vi "textParseController.vi"(8 "error in (no error)":errorcluster, 10 "file name":string, 11 "base path":path=path "C:/specsheetsController/Sheets/Controller") -> (0 "error out":errorcluster, 2 "all rows":string[][](array[string]), 3 "appended path":path)   [LabVIEW 2018]
uses:
  <vilib>/Utility/file.llb/Read Delimited Spreadsheet (string).vi
  Global textParse.vi
panel:
  out "protocolGrade":string
  out "protocolDistance":string
  out "protocolSpeed":string
  out "LED Frequency Max":string
  out "LED Frequency Min":string
  out "LED Frequency (Charge)":string
  out "LED Frequency (Limit)":string
  out "LED Frequency (Foldback)":string
  out "HV Bus Voltage(@10% PWM)":string
  out "HV Bus Tol. Min":string
  out "HV Bus Tol. Max":string
  out "Speed Pot Voltage Low(@85% PWM)":string
  out "Speed Pot Voltage Mid(@85% PWM)":string
  out "Speed Pot Voltage High(@85% PWM)":string
  out "Speed Pot Voltage Tol. Min":string
  out "Speed Pot Voltage Tol. Max":string
  out "Ircomp(@70% PWM)":string
  out "Current Running Tol. Min":string
  out "Current Running Tol. Max":string
  out "Current Limit(@45% PWM)":string
  out "Sense Voltage Tol. Max":string
  out "Sense Voltage Tol. Min":string
  out "Sense Voltage":string
  out "Allowable Power Interuption":string
  out "Voltage FET Driver Tol. Max":string
  out "Voltage FET Driver Tol. Min":string
  out "Voltage FET Driver":string
  out "Voltage Micro Tol. Max":string
  out "Voltage Micro Tol. Min":string
  out "Voltage Micro":string
  out "Rated Output Current Tol. Max":string
  out "Rated Output Current Tol. Min":string
  out "Rated Output Current":string
  out "Ripple/Noise Tol. Max":string
  out "Ripple/Noise Tol. Min":string
  out "Ripple/Noise":string
  out "Voltage Output Tol. Max":string
  out "Voltage  Output Tol. Min":string
  out "Voltage Output":string
  out "Max Input Current":string
  out "Input Current":string
  out "Input Voltage Tol. Max":string
  out "Input Voltage Tol. Min":string
  out "Input Voltage":string
  out "Firmware":string
  out "Part Number":string
  out "Part Name":string
  # "Global variables"
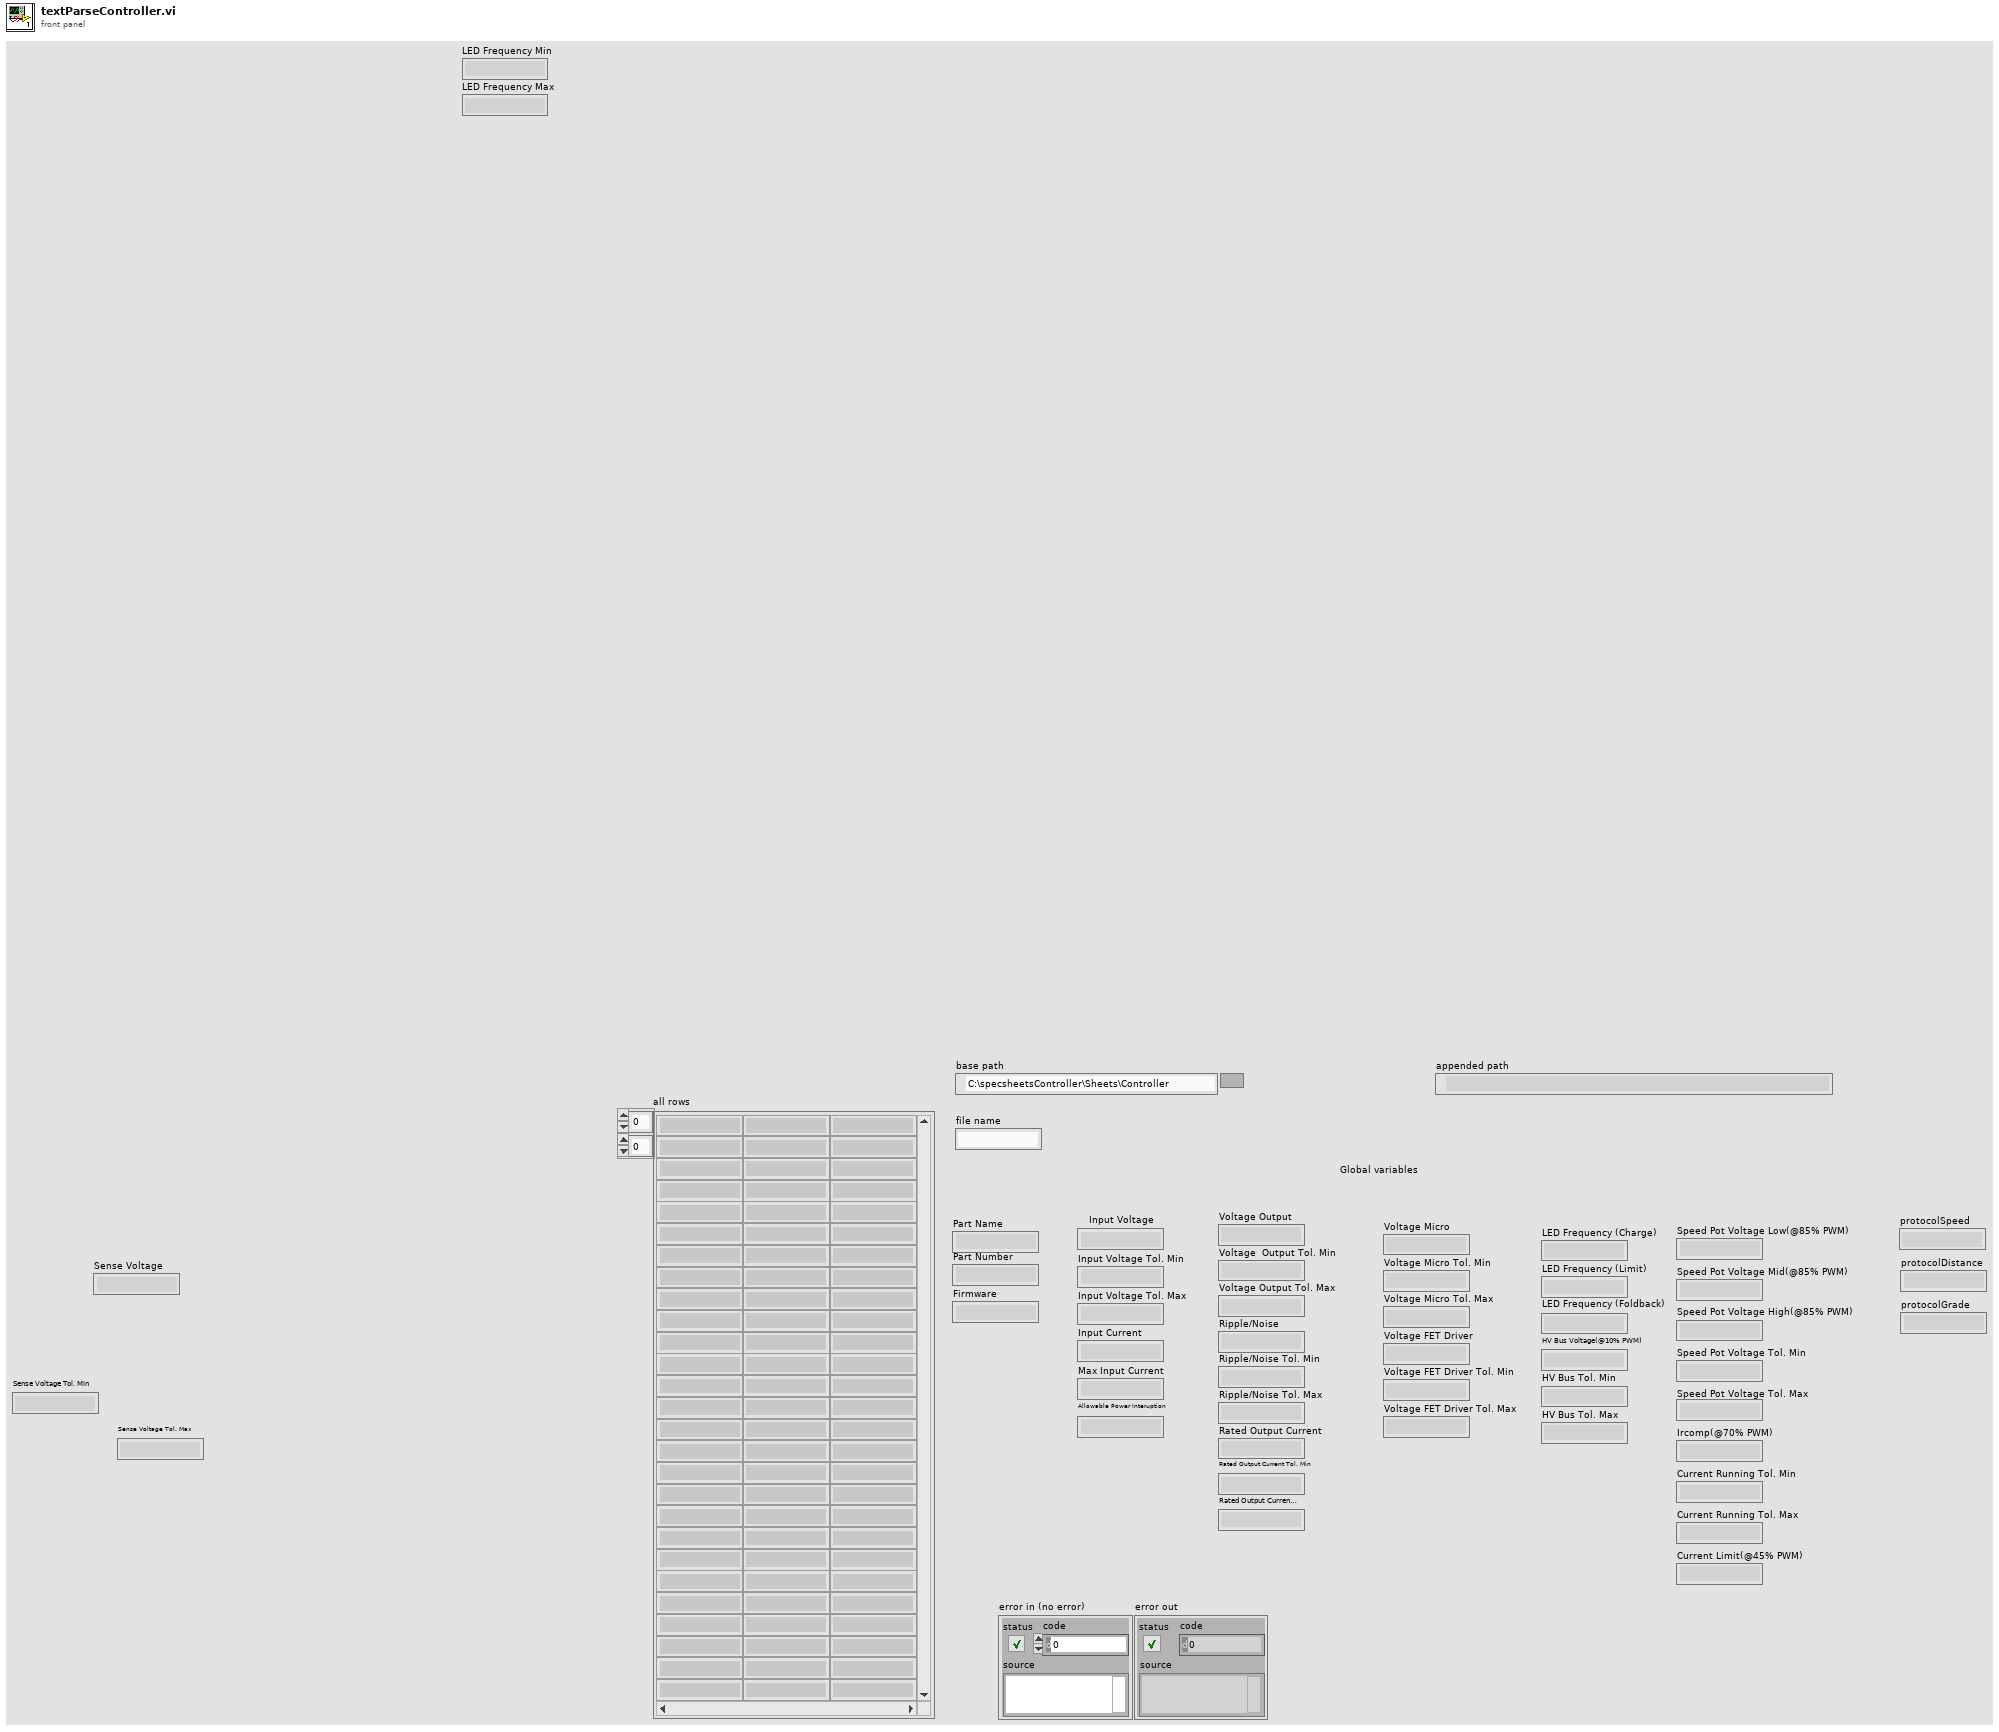
[diagram p1: front panel]
types:
  T1 = enum16{"Main", "In Primary", "Secondary", "Out Primary", "Motor Drive", "Protocol"}
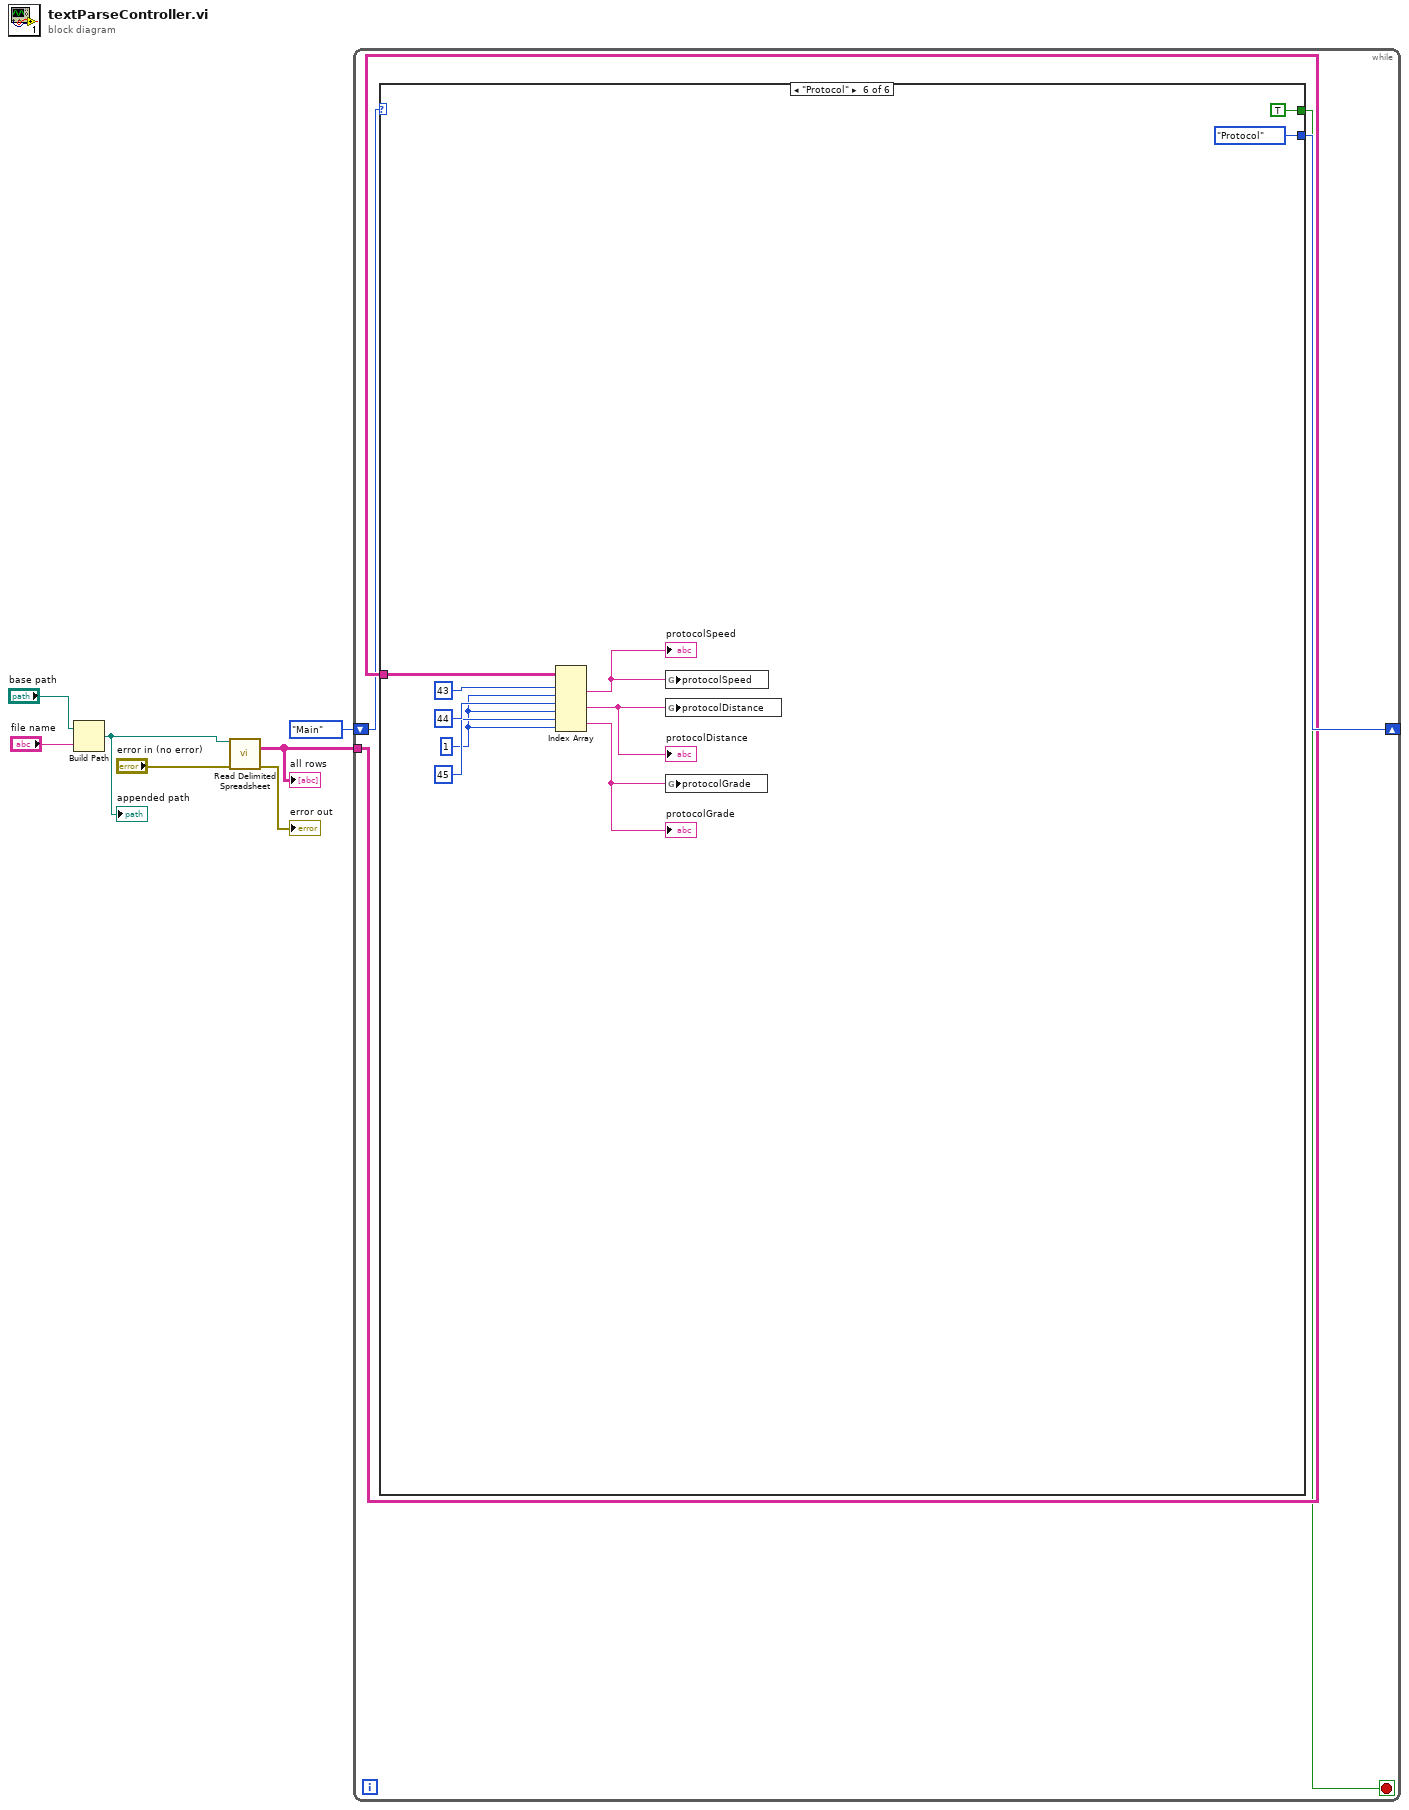
[diagram p0: block diagram]
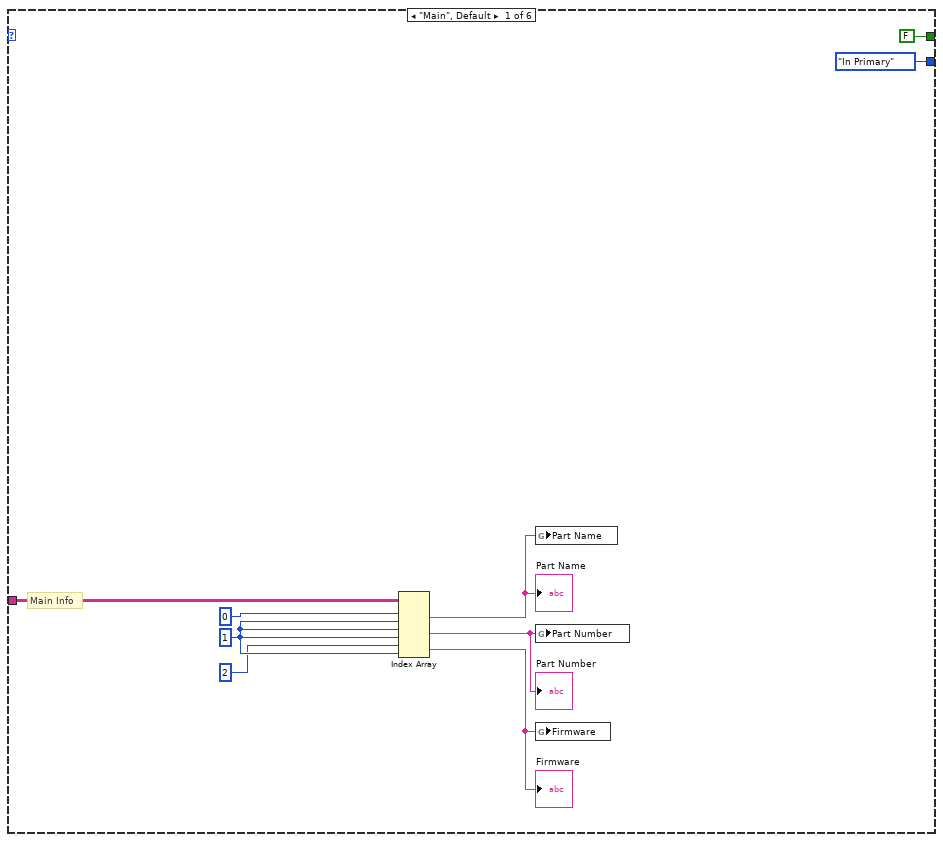
[diagram p2: hidden frame]
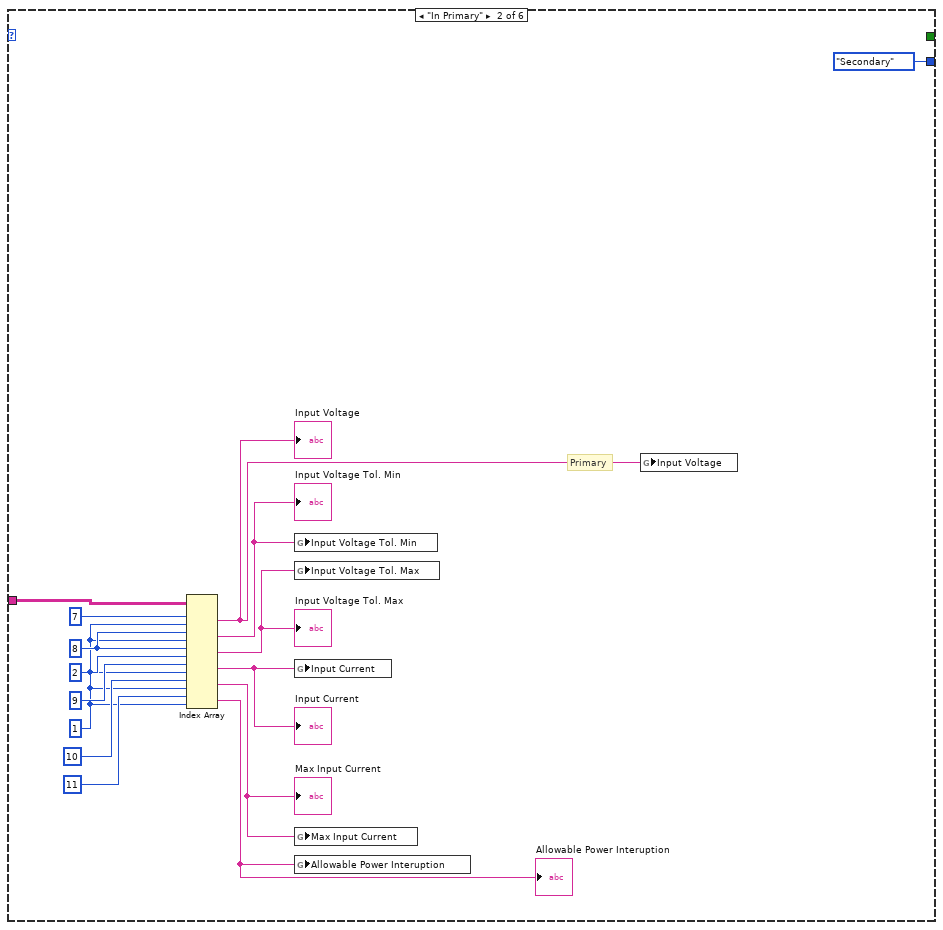
[diagram p3: hidden frame]
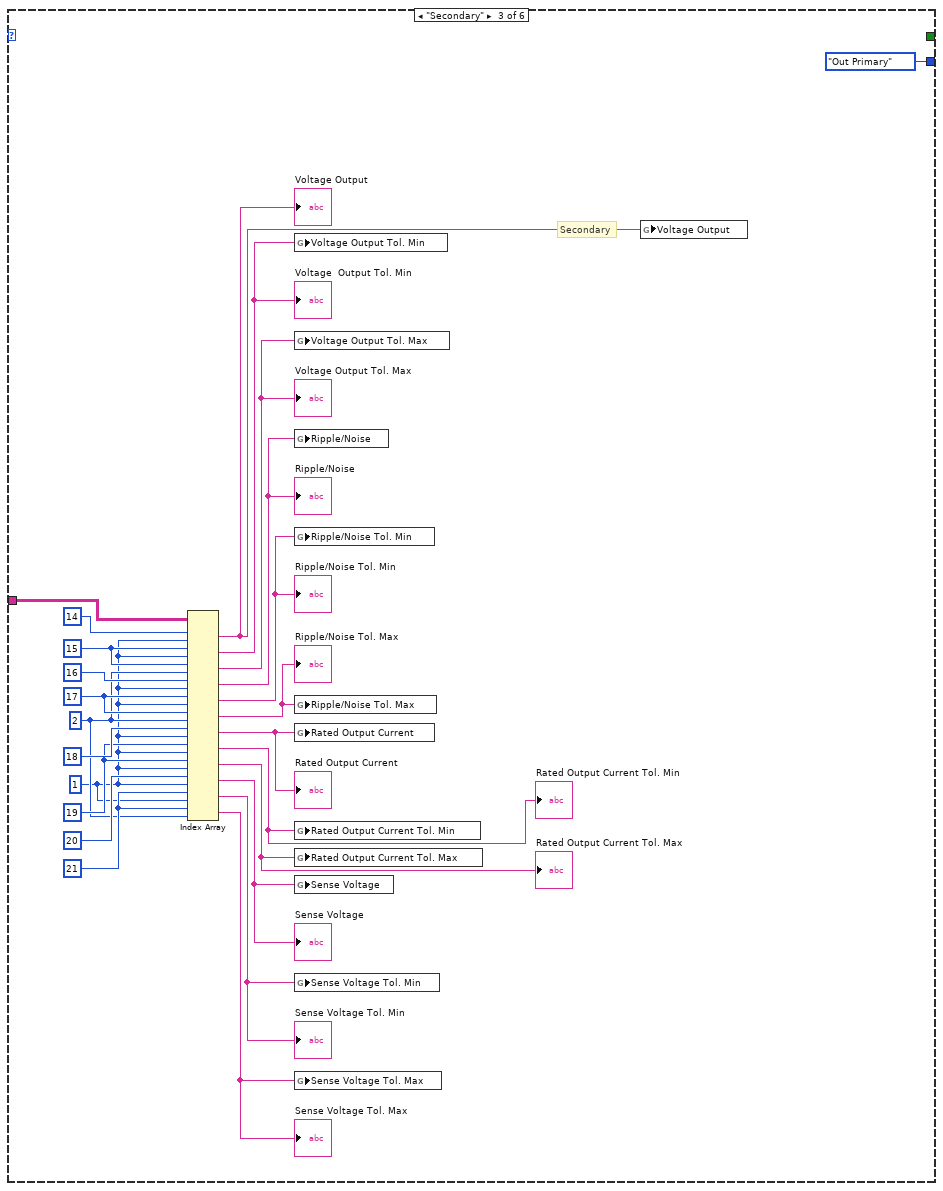
[diagram p4: hidden frame]
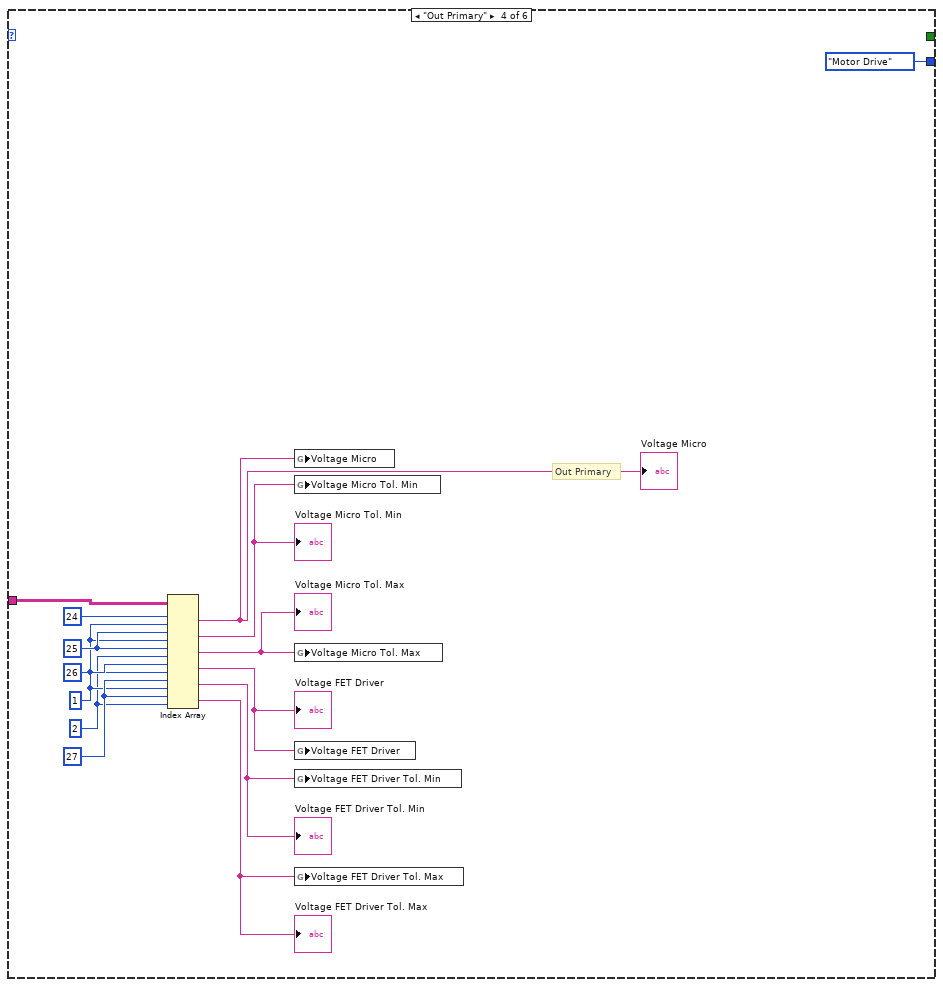
[diagram p5: hidden frame]
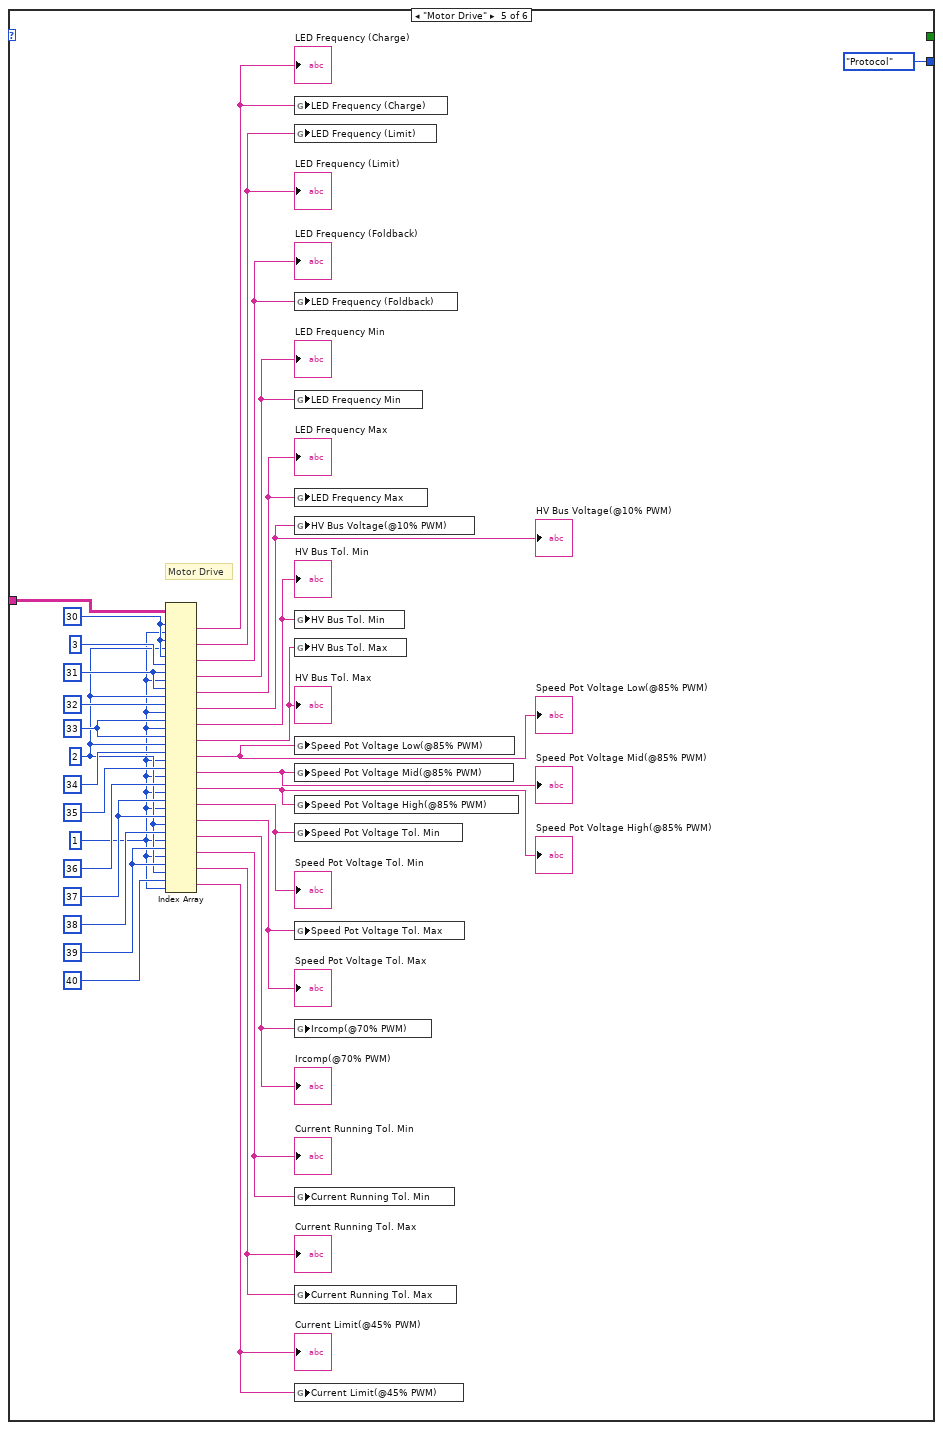
[diagram p6: hidden frame]
diagram:
  n1 = Build Path(base path="base path", name or relative path="file name") -> (appended path=w5:path)
  "appended path" <- w5
  n2 = call-poly <vilib>:"Read Delimited Spreadsheet.vi"("file path (dialog if empty)"=w5, "error in (no error)"="error in (no error)") -> ("all rows"=w2:string[][], "error out"=→"error out":errorcluster)  [unwired: 8 in, 4 out]
  "all rows" <- w2
  n3 = while {
    shift-right: [w11] -> _
    shift-left: T1."Main" -> [w9]
    tunnel: w2 -> [w10]
    stop <- w8 stop-if-true
    n4 = case shown="\"Protocol\"" w9 {
      tunnel: w10 -> [w14 w24 w44 w63 w106 w116]
      tunnel: [T1."In Primary" T1."Secondary" T1."Out Primary" T1."Motor Drive" T1."Protocol" T1."Protocol"] -> w11
      tunnel: [FALSE _ _ _ _ TRUE] -> w8
      frame "Main", Default {
        w16 = 1
        # "Main Info"
        n5 = Index Array(array=w14, index (row) #1=0 ("index (row)"), index (col) #1=w16, index (row) #2=w16, index (col) #2=w16, index (row) #3=2 ("index (row)"), index (col) #3=w16) -> (element #1=w18:string, element #2=w20:string, element #3=w19:string)
        "Part Name" <- w18
        "Part Number" <- w20
        "Firmware" <- w19
        n6 = global write "Global textParse.vi" "Part Name"(w18) -> ()
        n7 = global write "Global textParse.vi" "Part Number"(w20) -> ()
        n8 = global write "Global textParse.vi" "Firmware"(w19) -> ()
      }
      frame "In Primary" {
        w28 = 8
        w22 = 1
        # "Primary"
        n9 = Index Array(array=w24, index (row) #1=7, index (col) #1=w22, index (row) #2=w28, index (col) #2=w22, index (row) #3=w28, index (col) #3=2, index (row) #4=9, index (col) #4=w22, index (row) #5=10, index (col) #5=w22, index (row) #6=11, index (col) #6=w22) -> (element #1=w30:string, element #2=w31:string, element #3=w32:string, element #4=w33:string, element #5=w34:string, element #6=w35:string)
        "Input Voltage" <- w30
        "Input Voltage Tol. Min" <- w31
        "Input Voltage Tol. Max" <- w32
        "Input Current" <- w33
        "Max Input Current" <- w34
        "Allowable Power Interuption" <- w35
        n10 = global write "Global textParse.vi" "Input Voltage Tol. Min"(w31) -> ()
        n11 = global write "Global textParse.vi" "Input Voltage Tol. Max"(w32) -> ()
        n12 = global write "Global textParse.vi" "Input Current"(w33) -> ()
        n13 = global write "Global textParse.vi" "Max Input Current"(w34) -> ()
        n14 = global write "Global textParse.vi" "Allowable Power Interuption"(w35) -> ()
        n15 = global write "Global textParse.vi" "Input Voltage"(w30) -> ()
      }
      frame "Secondary" {
        w42 = 21 ("index (row)")
        w45 = 19 ("index (row)")
        w40 = 1
        w41 = 2
        w47 = 17 ("index (row) 15")
        w49 = 15 ("index (row) 13")
        # "Secondary"
        n16 = Index Array(array=w44, index (row) #1=14 ("index (row) 12"), index (col) #1=w40, index (row) #2=w49, index (col) #2=w40, index (row) #3=w49, index (col) #3=w41, index (row) #4=16 ("index (row) 14"), index (col) #4=w40, index (row) #5=w47, index (col) #5=w40, index (row) #6=w47, index (col) #6=w41, index (row) #7=18 ("index (row) 19"), index (col) #7=w40, index (row) #8=w45, index (col) #8=w40, index (row) #9=w45, index (col) #9=w40, index (row) #10=20 ("index (row)"), index (col) #10=w40, index (row) #11=w42, index (col) #11=w40, index (row) #12=w42, index (col) #12=w41) -> (element #1=w51:string, element #2=w52:string, element #3=w53:string, element #4=w54:string, element #5=w55:string, element #6=w56:string, element #7=w57:string, element #8=w58:string, element #9=w59:string, element #10=w39:string, element #11=w38:string, element #12=w37:string)
        "Voltage Output" <- w51
        "Voltage  Output Tol. Min" <- w52
        "Voltage Output Tol. Max" <- w53
        "Ripple/Noise" <- w54
        "Ripple/Noise Tol. Min" <- w55
        "Ripple/Noise Tol. Max" <- w56
        "Rated Output Current" <- w57
        "Rated Output Current Tol. Min" <- w58
        "Rated Output Current Tol. Max" <- w59
        "Sense Voltage" <- w39
        "Sense Voltage Tol. Min" <- w38
        "Sense Voltage Tol. Max" <- w37
        n17 = global write "Global textParse.vi" "Voltage Output Tol. Min"(w52) -> ()
        n18 = global write "Global textParse.vi" "Voltage Output Tol. Max"(w53) -> ()
        n19 = global write "Global textParse.vi" "Ripple/Noise"(w54) -> ()
        n20 = global write "Global textParse.vi" "Ripple/Noise Tol. Min"(w55) -> ()
        n21 = global write "Global textParse.vi" "Ripple/Noise Tol. Max"(w56) -> ()
        n22 = global write "Global textParse.vi" "Rated Output Current"(w57) -> ()
        n23 = global write "Global textParse.vi" "Rated Output Current Tol. Min"(w58) -> ()
        n24 = global write "Global textParse.vi" "Rated Output Current Tol. Max"(w59) -> ()
        n25 = global write "Global textParse.vi" "Sense Voltage"(w39) -> ()
        n26 = global write "Global textParse.vi" "Sense Voltage Tol. Min"(w38) -> ()
        n27 = global write "Global textParse.vi" "Sense Voltage Tol. Max"(w37) -> ()
        n28 = global write "Global textParse.vi" "Voltage Output"(w51) -> ()
      }
      frame "Out Primary" {
        w61 = 2
        w62 = 1
        w64 = 27 ("index (row) 27")
        w66 = 25 ("index (row) 25")
        # "Out Primary"
        n29 = Index Array "Index Array"(array=w63, index (row) #1=24 ("index (row) 24"), index (col) #1=w62, index (row) #2=w66, index (col) #2=w62, index (row) #3=w66, index (col) #3=w61, index (row) #4=26 ("index (row) 26"), index (col) #4=w62, index (row) #5=w64, index (col) #5=w62, index (row) #6=w64, index (col) #6=w61) -> (element #1=w68:string, element #2=w69:string, element #3=w70:string, element #4=w71:string, element #5=w72:string, element #6=w73:string)
        "Voltage Micro" <- w68
        "Voltage Micro Tol. Min" <- w69
        "Voltage Micro Tol. Max" <- w70
        "Voltage FET Driver" <- w71
        "Voltage FET Driver Tol. Min" <- w72
        "Voltage FET Driver Tol. Max" <- w73
        n30 = global write "Global textParse.vi" "Voltage Micro"(w68) -> ()
        n31 = global write "Global textParse.vi" "Voltage Micro Tol. Min"(w69) -> ()
        n32 = global write "Global textParse.vi" "Voltage Micro Tol. Max"(w70) -> ()
        n33 = global write "Global textParse.vi" "Voltage FET Driver"(w71) -> ()
        n34 = global write "Global textParse.vi" "Voltage FET Driver Tol. Min"(w72) -> ()
        n35 = global write "Global textParse.vi" "Voltage FET Driver Tol. Max"(w73) -> ()
      }
      frame "Motor Drive" {
        w93 = 2
        w92 = 1
        w95 = 39
        w97 = 37
        w101 = 33 ("index (row) 28")
        w103 = 31 ("index (row) 25")
        w104 = 30 ("index (row) 24")
        # "Motor Drive"
        n36 = Index Array "Index Array"(array=w106, index (row) #1=w104, index (col) #1=w92, index (row) #2=w104, index (col) #2=w93, index (row) #3=w104, index (col) #3=3, index (row) #4=w103, index (col) #4=w92, index (row) #5=w103, index (col) #5=w93, index (row) #6=32 ("index (row) 26"), index (col) #6=w92, index (row) #7=w101, index (col) #7=w92, index (row) #8=w101, index (col) #8=w93, index (row) #9=34 ("index (row) 29"), index (col) #9=w92, index (row) #10=35, index (col) #10=w92, index (row) #11=36 ("index (row) 30"), index (col) #11=w92, index (row) #12=w97, index (col) #12=w92, index (row) #13=w97, index (col) #13=w93, index (row) #14=38, index (col) #14=w92, index (row) #15=w95, index (col) #15=w92, index (row) #16=w95, index (col) #16=w93, index (row) #17=40, index (col) #17=w92) -> (element #1=w91:string, element #2=w90:string, element #3=w89:string, element #4=w88:string, element #5=w87:string, element #6=w86:string, element #7=w85:string, element #8=w84:string, element #9=w83:string, element #10=w82:string, element #11=w81:string, element #12=w80:string, element #13=w79:string, element #14=w78:string, element #15=w77:string, element #16=w76:string, element #17=w75:string)
        "LED Frequency (Charge)" <- w91
        "LED Frequency (Limit)" <- w90
        "LED Frequency (Foldback)" <- w89
        "HV Bus Voltage(@10% PWM)" <- w86
        "HV Bus Tol. Min" <- w85
        "HV Bus Tol. Max" <- w84
        "Speed Pot Voltage Low(@85% PWM)" <- w83
        "Speed Pot Voltage Mid(@85% PWM)" <- w82
        "Speed Pot Voltage High(@85% PWM)" <- w81
        "Speed Pot Voltage Tol. Min" <- w80
        "Speed Pot Voltage Tol. Max" <- w79
        "Ircomp(@70% PWM)" <- w78
        "Current Running Tol. Min" <- w77
        "Current Running Tol. Max" <- w76
        "Current Limit(@45% PWM)" <- w75
        "LED Frequency Min" <- w88
        "LED Frequency Max" <- w87
        n37 = global write "Global textParse.vi" "LED Frequency (Charge)"(w91) -> ()
        n38 = global write "Global textParse.vi" "LED Frequency (Limit)"(w90) -> ()
        n39 = global write "Global textParse.vi" "LED Frequency (Foldback)"(w89) -> ()
        n40 = global write "Global textParse.vi" "LED Frequency Min"(w88) -> ()
        n41 = global write "Global textParse.vi" "LED Frequency Max"(w87) -> ()
        n42 = global write "Global textParse.vi" "HV Bus Voltage(@10% PWM)"(w86) -> ()
        n43 = global write "Global textParse.vi" "HV Bus Tol. Min"(w85) -> ()
        n44 = global write "Global textParse.vi" "HV Bus Tol. Max"(w84) -> ()
        n45 = global write "Global textParse.vi" "Speed Pot Voltage Low(@85% PWM)"(w83) -> ()
        n46 = global write "Global textParse.vi" "Speed Pot Voltage Mid(@85% PWM)"(w82) -> ()
        n47 = global write "Global textParse.vi" "Speed Pot Voltage High(@85% PWM)"(w81) -> ()
        n48 = global write "Global textParse.vi" "Speed Pot Voltage Tol. Min"(w80) -> ()
        n49 = global write "Global textParse.vi" "Speed Pot Voltage Tol. Max"(w79) -> ()
        n50 = global write "Global textParse.vi" "Ircomp(@70% PWM)"(w78) -> ()
        n51 = global write "Global textParse.vi" "Current Running Tol. Min"(w77) -> ()
        n52 = global write "Global textParse.vi" "Current Running Tol. Max"(w76) -> ()
        n53 = global write "Global textParse.vi" "Current Limit(@45% PWM)"(w75) -> ()
      }
      frame "Protocol" {
        w112 = 1 ("disabled index (col)")
        n54 = Index Array(array=w116, index (row) #1=43 ("index (row)"), index (col) #1=w112, index (row) #2=44 ("index (row)"), index (col) #2=w112, index (row) #3=45 ("index (row)"), index (col) #3=w112) -> (element #1=w107:string, element #2=w108:string, element #3=w109:string)
        "protocolSpeed" <- w107
        "protocolDistance" <- w108
        "protocolGrade" <- w109
        n55 = global write "Global textParse.vi" "protocolSpeed"(w107) -> ()
        n56 = global write "Global textParse.vi" "protocolDistance"(w108) -> ()
        n57 = global write "Global textParse.vi" "protocolGrade"(w109) -> ()
      }
    }
  }
